vi "Xeryon unit conversion.vi"(3 "Type":T1, 4 "Value in":dbl, 5 "Mode":T2(ring)) -> (1 "Value out":dbl)   [LabVIEW 2019]
uses:
  Axis Manager/Axis enum.ctl
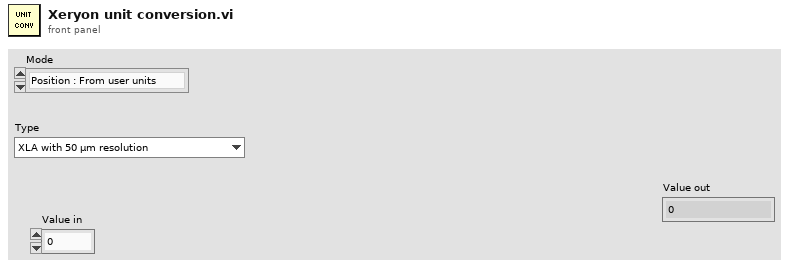
[diagram p1: front panel]
types:
  T1 = typedef "Axis enum.ctl" = enum16{"XLA with 50 µm resolution", "XLA with 10 µm resolution", "XLA with 1250 nm resolution", "XLA with 312 nm resolution", "XLA with 78 nm resolution", "XLS with 1250 nm resolution", "XLS with 312 nm resolution", "XLS with 78nm resolution", "XLS with 5nm resolution", "XLS with 1 nm resolution", "XRT-A with 109 µrad resolution", "XRT-U-30 with 109 µrad resolution", "XRT-U-30 with 49 µrad resolution", "XRT-U-30 with 19 µrad resolution", "XRT-U-30 with 3 µrad resolution", "XRT-U-40 with 109 µrad resolution", "XRT-U 40 with 49 µrad resolution", "XRT-U-40 with 19 µrad resolution", "XRT-U-40 with 3 µrad resolution", "XRT-U-60 with 109 µrad resolution", "XRT-U-60 with 49 µrad resolution", "XRT-U-60 with 19 µrad resolution", "XRT-U-60 with 3 µrad resolution"}
  T2 = enum16{"Position : From user units", "Position : To user units"}
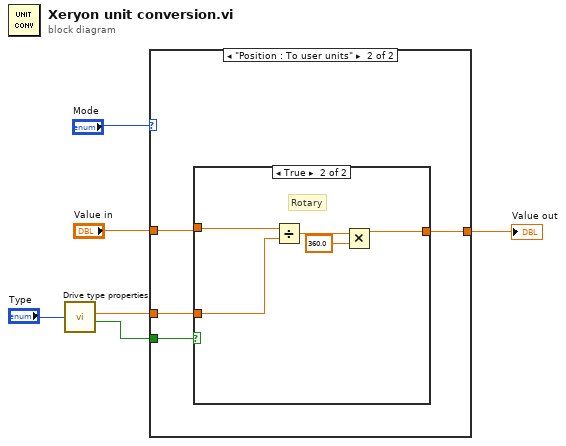
[diagram p0: block diagram]
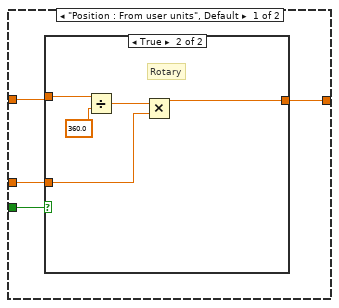
[diagram p2: hidden frame]
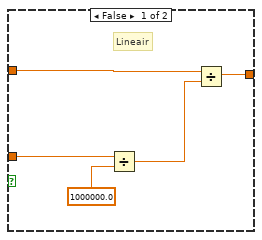
[diagram p3: hidden frame]
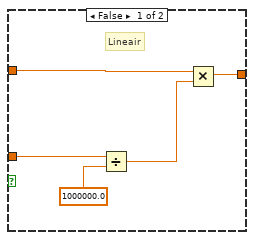
[diagram p4: hidden frame]
diagram:
  n1 = call "Drive type properties.vi"("Type"="Type") -> ("Effective resolution"=w2:dbl, "Rotary"=w1:bool)  [unwired: 2 in, 2 out]
  n2 = case shown="\"Position : To user units\"" "Mode" {
    tunnel: "Value in" -> [w10 w24]
    tunnel: [w7 w21] -> w4
    tunnel: w2 -> [w9 w23]
    tunnel: w1 -> [w8 w22]
    frame "Position : From user units", Default {
      n3 = case shown="True" w8 {
        tunnel: w10 -> [w15 w19]
        tunnel: w9 -> [w13 w20]
        tunnel: [w11 w16] -> w7
        frame False {
          # "Lineair"
          n4 = Divide(x=w13, y=1000000.0) -> (x/y=w12:dbl)
          n5 = Divide(x=w15, y=w12) -> (x/y=w11:dbl)
        }
        frame True {
          # "Rotary"
          n6 = Divide(x=w19, y=360.0) -> (x/y=w17:dbl)
          n7 = Multiply(x=w17, y=w20) -> (x*y=w16:dbl)
        }
      }
    }
    frame "Position : To user units" {
      n8 = case shown="True" w22 {
        tunnel: w24 -> [w29 w34]
        tunnel: w23 -> [w27 w33]
        tunnel: [w25 w30] -> w21
        frame False {
          # "Lineair"
          n9 = Divide(x=w27, y=1000000.0) -> (x/y=w26:dbl)
          n10 = Multiply(x=w29, y=w26) -> (x*y=w25:dbl)
        }
        frame True {
          # "Rotary"
          n11 = Divide(x=w34, y=w33) -> (x/y=w32:dbl)
          n12 = Multiply(x=w32, y=360.0) -> (x*y=w30:dbl)
        }
      }
    }
  }
  "Value out" <- w4
